vi "Vision Target.vi"() -> ()   [LabVIEW 2018]
uses:
  Vision/Camera Types.ctl
  <vilib>/vision/NI_Vision_Development_Module.lvlib
panel:
  out "Distance (ft)":dbl
  out "Angle":dbl
  out "Image 3":T1(plugin-control)
  out "Particles":i32
  out "Image":T1(plugin-control)
  in  "Image":path
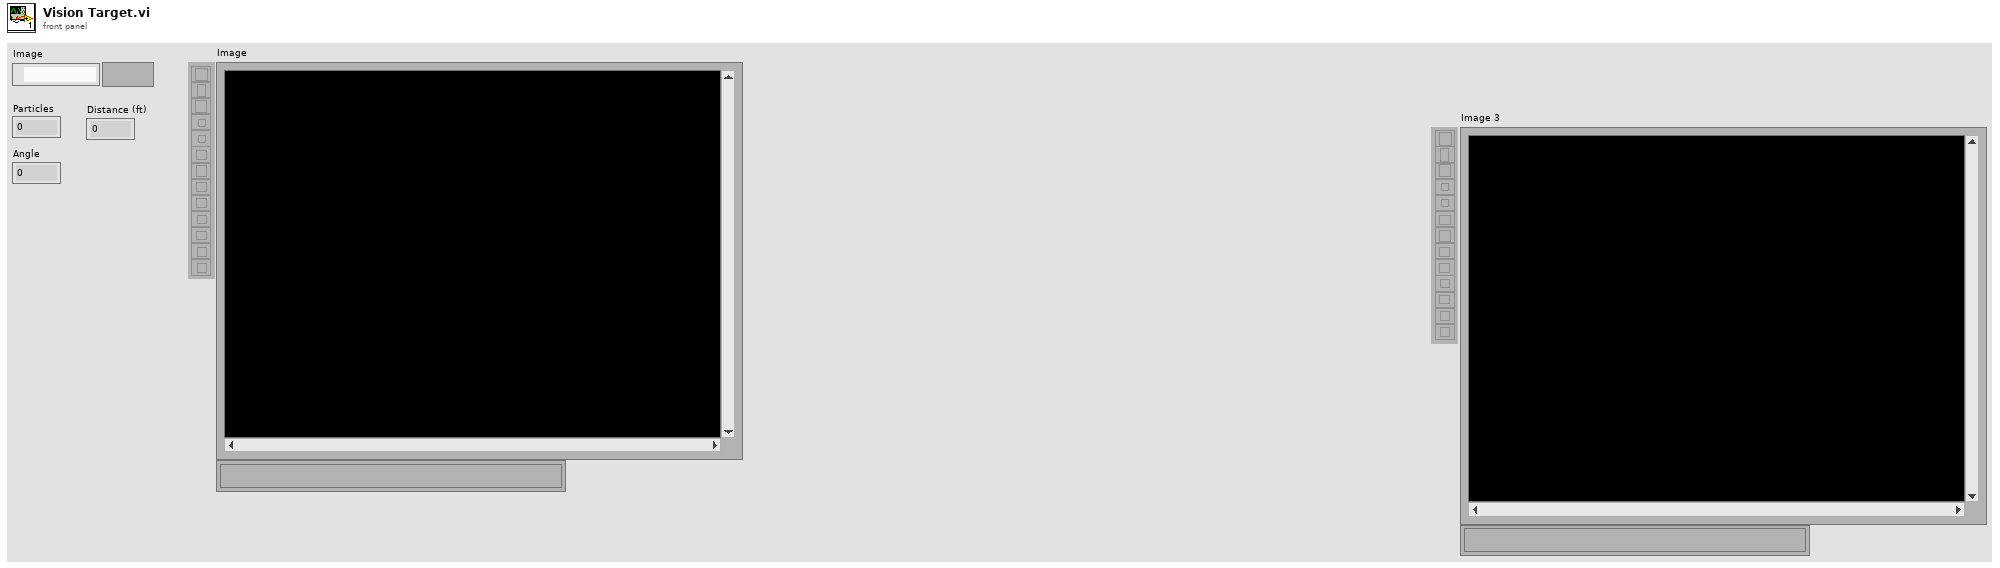
[diagram p1: front panel]
types:
  T1 = typedef "IMAQ Image.ctl" = refnum<image>
  T2 = typedef "Particle Parameters" = i32
  T3 = typedef "Image Type" = u32
  T4 = typedef "Camera Types.ctl" = enum16{"206", "1011", "1013", "MS HD3000 square", "MS HD3000 640x480"}
  T5 = cluster{"Score":dbl, "Rect":cluster{"Left":dbl, "Top":dbl, "Right":dbl, "Bottom":dbl}, "Full Scores":cluster{"Aspect Ratio":dbl, "Top Position":dbl, "Bottom Position":dbl, "Left Gap":dbl, "Width":dbl, "Height Ratio":dbl, "Angle":dbl}}[]
  T6 = cluster{"Score":dbl, "Rect":cluster{"Left":dbl, "Top":dbl, "Right":dbl, "Bottom":dbl}, "Full Scores":cluster{"Aspect Ratio":dbl, "Top Position":dbl, "Bottom Position":dbl, "Left Gap":dbl, "Width":dbl, "Height Ratio":dbl, "Angle":dbl}}
  T7 = cluster{"Left":dbl, "Top":dbl, "Right":dbl, "Bottom":dbl}
  T8 = cluster{"Numeric":dbl, "Numeric":dbl, "Numeric":dbl, "Numeric":dbl}
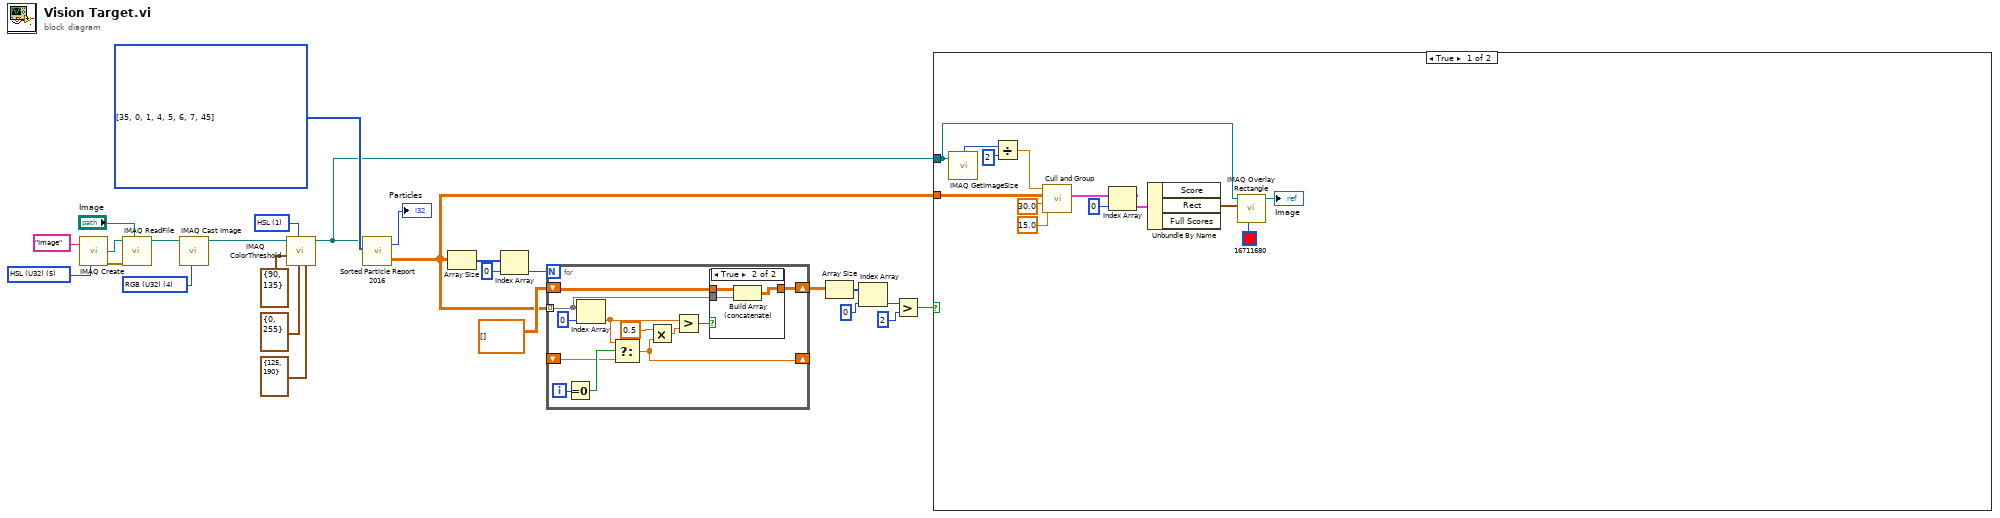
[diagram p0: block diagram]
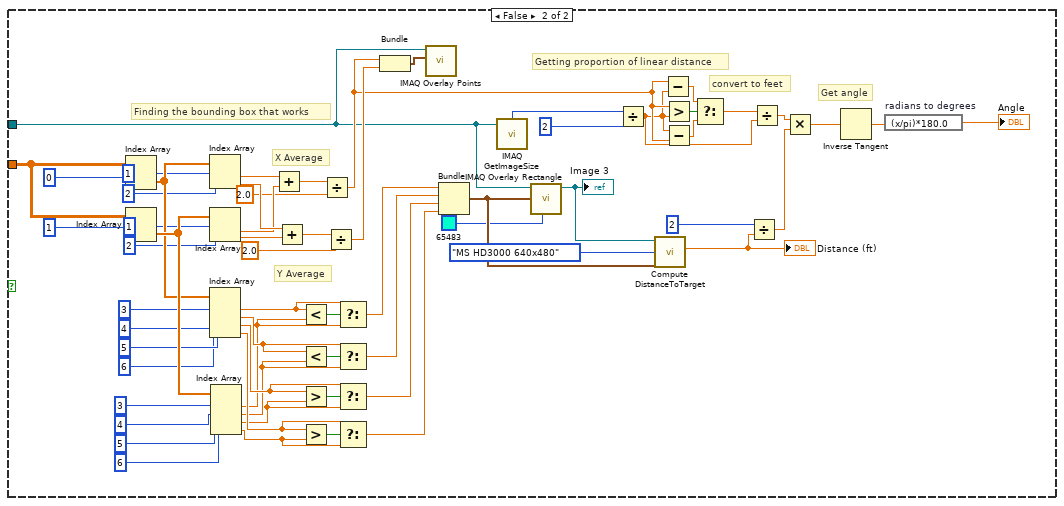
[diagram p2: hidden frame]
diagram:
  w14 = T2[] [35, 0, 1, 4, 5, 6, 7, 45] items=["Center of Mass X", "Center of Mass Y", "First Pixel X", "First Pixel Y", "Bounding Rect Left", "Bounding Rect Top", "Bounding Rect Right", "Bounding Rect Bottom", "Max Feret Diameter Start X", "Max Feret Diameter Start Y", "Max Feret Diameter End X", "Max Feret Diameter End Y", "Max Horiz. Segment Length Left", "Max Horiz. Segment Length Right", "Max Horiz. Segment Length Row", "-", "Bounding Rect Width", "Bounding Rect Height", "Bounding Rect Diagonal", "Perimeter", "Convex Hull Perimeter", "Holes' Perimeter", "Max Feret Diameter", "Equivalent Ellipse Major Axis", "Equivalent Ellipse Minor Axis", "Equivalent Ellipse Minor Axis (Feret)", "Equivalent Rect Long Side", "Equivalent Rect Short Side", "Equivalent Rect Diagonal", "Equivalent Rect Short Side (Feret)", "Average Horiz. Segment Length", "Average Vert. Segment Length", "Hydraulic Radius", "Waddel Disk Diameter", "-", "Area", "Holes' Area", "Particle & Holes' Area", "Convex Hull Area", "Image Area", "-", "Number of Holes", "Number of Horiz. Segments", "Number of Vert. Segments", "-", "Orientation", "Max Feret Diameter Orientation", "-", "% Area/Image Area", "% Area/(Particle & Holes' Area)", "Ratio of Equivalent Ellipse Axes", "Ratio of Equivalent Rect Sides", "-", "Elongation Factor", "Compactness Factor", "Heywood Circularity Factor", "Type Factor", "-", "Sum X", "Sum Y", "Sum XX", "Sum XY", "Sum YY", "Sum XXX", "Sum XXY", "Sum XYY", "Sum YYY", "-", "Moment of Inertia XX", "Moment of Inertia XY", "Moment of Inertia YY", "Moment of Inertia XXX", "Moment of Inertia XXY", "Moment of Inertia XYY", "Moment of Inertia YYY", "Norm. Moment of Inertia XX", "Norm. Moment of Inertia XY", "Norm. Moment of Inertia YY", "Norm. Moment of Inertia XXX", "Norm. Moment of Inertia XXY", "Norm. Moment of Inertia XYY", "Norm. Moment of Inertia YYY", "Hu Moment 1", "Hu Moment 2", "Hu Moment 3", "Hu Moment 4", "Hu Moment 5", "Hu Moment 6", "Hu Moment 7"] ("Pixel Measurements")
  w16 = T3 5 items=["Grayscale (U8)", "Grayscale (I16)", "Grayscale (SGL)", "Complex (CSG)", "RGB (U32)", "HSL (U32)", "RGB (U64)", "Grayscale (U16)"] ("Image Type")
  w18 = T3 4 items=["Grayscale (U8)", "Grayscale (I16)", "Grayscale (SGL)", "Complex (CSG)", "RGB (U32)", "HSL (U32)", "RGB (U64)", "Grayscale (U16)"] ("Image Type")
  w22 = u16 1 items=["RGB", "HSL", "HSV", "HSI"] ("Color Mode")
  n1 = call "IMAQ Create"("Image Name"="Image", "Image Type"=w16) -> ("New Image"=w25:T1, "error out"=w26:errorcluster)  [unwired: 3 in]
  n2 = call "IMAQ ReadFile"("File Path"="Image", "error in (no error)"=w26, "Image"=w25) -> ("Image Out"=w17:T1)  [unwired: 4 in, 4 out]
  n3 = call "IMAQ Cast Image"("Image Type"=w18, "Image Src"=w17) -> ("Image Dst Out"=w2:T1)  [unwired: 8 in, 1 out]
  n4 = call "IMAQ ColorThreshold"("Blue or Luma or Val or Inten Range"=cluster{"Lower value":i32, "Upper value":i32} {"Lower value"=125, "Upper value"=190}, "Green or Sat Range"=cluster{"Lower value":i32, "Upper value":i32} {"Lower value"=0, "Upper value"=255}, "Color Mode"=w22, "Red or Hue Range"=cluster{"Lower value":i32, "Upper value":i32} {"Lower value"=90, "Upper value"=135}, "Image Src"=w2) -> ("Image Dst Out"=w1:T1)  [unwired: 5 in, 1 out]
  n5 = call "Sorted Particle Report 2016.vi"("Pixel Measurements"=w14, "Image in"=w1) -> ("Sorted Data"=w3:dbl[][], "Particles"=→"Particles":i32)  [unwired: 2 in]
  n6 = Array Size(array=w3) -> (size(s)=w8:i32[])
  n7 = Index Array(array=w8, index=0) -> (element=w6:i32)
  n8 = for {
    N: w6 -> [_]
    tunnel: w3 -> [w30] mode=indexing
    shift-right: [w34] -> _
    shift-left: _ -> [w35]
    shift-right: [w28] -> w5
    shift-left: dbl[][] [] -> [w29]
    i -> [w38]
    n9 = Equal To 0?(x=w38) -> (x = 0?=w36:bool)
    n10 = Index Array(array=w30, index=0) -> (element=w31:dbl)
    n11 = Select(t=w31, s=w36, f=w35) -> (s? t:f=w34:dbl)
    n12 = Multiply(x=0.5, y=w34) -> (x*y=w32:dbl)
    n13 = Greater?(x=w31, y=w32) -> (0:w27:bool)
    n14 = case shown="True" w27 {
      tunnel: w30 -> [_ w42]
      tunnel: w29 -> [w39 w41]
      tunnel: [w39 w40] -> w28
      frame False {
      }
      frame True {
        n15 = Build Array (concatenate)(w41, w42) -> (w40:dbl[][])
      }
    }
  }
  n16 = Array Size(array=w5) -> (size(s)=w11:i32[])
  n17 = Index Array(array=w11, index=0 ("y")) -> (element=w9:i32)
  n18 = Greater?(x=w9, y=2) -> (0:w4:bool)
  n19 = case shown="True" w4 {
    tunnel: w1 -> [w43 w57]
    tunnel: w3 -> [w51 w56]
    frame True {
      n20 = call "IMAQ GetImageSize"("Image"=w43) -> ("X Resolution"=w46:i32)  [unwired: 3 in, 2 out]
      n21 = Divide(x=w46, y=2) -> (x/y=w44:dbl)
      n22 = call "Cull and Group.vi"("Min Compnt %"=15.0, "Score Cutoff %"=30.0, "Sorted Data"=w51, "Image Center"=w44) -> ("Best Targets above cutoff"=w55:T5)  [unwired: 7 in]
      n23 = Index Array(array=w55, index=0) -> (element=w53:T6)
      n24 = Unbundle By Name(w53) -> ("Rect"=w52:T7)  [unwired: 2 out]
      n25 = call "IMAQ Overlay Rectangle"("Color"=u32 16711680, "Rectangle"=w52, "Image"=w43) -> ("Image Out"=→"Image":T1)  [unwired: 7 in, 1 out]
    }
    frame False {
      # "convert to feet"
      # "Get angle"
      # "Getting proportion of linear distance"
      # "Finding the bounding box that works"
      # "Y Average"
      # "X Average"
      n26 = Index Array(array=w56, index (row)=0) -> (element=w95:dbl[])  [unwired: 1 in]
      n27 = Index Array(array=w56, index (row)=1 ("disabled index (col)")) -> (element=w96:dbl[])  [unwired: 1 in]
      n28 = Index Array(array=w95, index #1=1 ("index"), index #2=2 ("index")) -> (element #1=w81:dbl, element #2=w83:dbl)
      n29 = Index Array(array=w96, index #1=1 ("index"), index #2=2 ("index")) -> (element #1=w82:dbl, element #2=w80:dbl)
      n30 = Index Array(array=w95, index #1=3 ("index"), index #2=4 ("index"), index #3=5 ("index"), index #4=6 ("index")) -> (element #1=w98:dbl, element #2=w102:dbl, element #3=w104:dbl, element #4=w107:dbl)
      n31 = Index Array(array=w96, index #1=3 ("index"), index #2=4 ("index"), index #3=5 ("index"), index #4=6 ("index")) -> (element #1=w99:dbl, element #2=w101:dbl, element #3=w105:dbl, element #4=w108:dbl)
      n32 = Add(x=w81, y=w82) -> (x+y=w78:dbl)
      n33 = Add(x=w83, y=w80) -> (x+y=w79:dbl)
      n34 = Less?(x=w98, y=w99) -> (x < y?=w97:bool)
      n35 = Less?(x=w102, y=w101) -> (x < y?=w100:bool)
      n36 = Greater?(x=w104, y=w105) -> (0:w103:bool)
      n37 = Greater?(x=w107, y=w108) -> (0:w106:bool)
      n38 = Divide(x=w78, y=2.0) -> (x/y=w115:dbl)
      n39 = Divide(x=w79, y=2.0) -> (x/y=w116:dbl)
      n40 = Select(t=w98, s=w97, f=w99) -> (s? t:f=w109:dbl)
      n41 = Select(t=w102, s=w100, f=w101) -> (s? t:f=w110:dbl)
      n42 = Select(t=w104, s=w103, f=w105) -> (s? t:f=w111:dbl)
      n43 = Select(t=w107, s=w106, f=w108) -> (s? t:f=w112:dbl)
      n44 = Bundle(w115, w116) -> (w114:cluster{dbl, dbl})  [unwired: 1 in]
      n45 = call "IMAQ Overlay Points"("Point"=w114, "Image"=w57) -> ()  [unwired: 8 in, 2 out]
      n46 = Bundle("Numeric"=w109, "Numeric"=w110, "Numeric"=w111, "Numeric"=w112) -> (w113:T8)  [unwired: 1 in]
      n47 = call "IMAQ GetImageSize"("Image"=w57) -> ("X Resolution"=w84:i32)  [unwired: 3 in, 2 out]
      n48 = call "IMAQ Overlay Rectangle"("Color"=u32 65483, "Rectangle"=w113, "Image"=w57) -> ("Image Out"=w94:T1)  [unwired: 7 in, 1 out]
      "Image 3" <- w94
      n49 = Divide(x=w84, y=2) -> (x/y=w93:dbl)
      n50 = call "Compute DistanceToTarget.vi"("Rect"=w113, "Camera Type"=Camera_Types."MS HD3000 640x480", "Image Src"=w94) -> ("Distance (ft)"=w117:dbl)  [unwired: 7 in, 1 out]
      "Distance (ft)" <- w117
      n51 = Subtract(x=w115, y=w93) -> (x-y=w86:dbl)
      n52 = Greater?(x=w115, y=w93) -> (0:w85:bool)
      n53 = Subtract(x=w93, y=w115) -> (x-y=w92:dbl)
      n54 = Select(t=w86, s=w85, f=w92) -> (s? t:f=w89:dbl)
      n55 = Divide(x=2, y=w117) -> (x/y=w118:dbl)
      n56 = Divide(x=w89, y=w93) -> (x/y=w90:dbl)
      n57 = Multiply(x=w90, y=w118) -> (x*y=w91:dbl)
      n58 = Inverse Tangent(1:w91) -> (0:w87:dbl)
      n59 = expression code="(x/pi)*180.0" "radians to degrees"(w87) -> (→"Angle":dbl)
    }
  }
